vi "PH_Beckhoff_PP_PU.set RR GUI Elements to Default.vi"(0 "i ref in":refnum<vi>, 2 "PUs":T2[](array[typedef]), 5 "error in":errorcluster) -> (14 "i ref out":refnum<vi>, 19 "error out":errorcluster)   [LabVIEW 2014, in "PH_Beckhoff_PP_PU.lvlib"]
uses:
  PH_Beckhoff_PP_PU.lvlib
  PH_Basics/PH_PP_Common/PH_PP_Common.PUs.ctl
  PH_Beckhoff_PP_PU.RR Tags.ctl
  PH_Basics/PH_Common/Names/PH_Names.Subsystems.ctl
  PH_Basics/PH_PP_Common/PH_PP_Common.Devices.ctl
  PH_Basics/PH_Common/PH_Common.lvlib
  PH_Basics/PH_PP_Common/PH_PP_Common.lvlib
panel:
  in  "Ross Relais Tags":T1
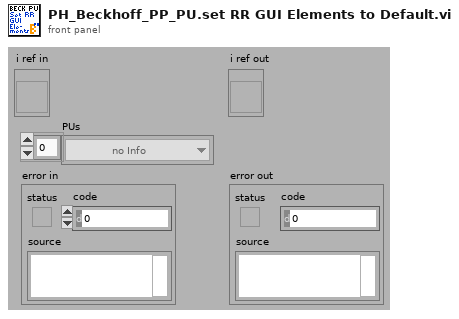
[diagram p1: front panel]
types:
  T1 = typedef "PH_Beckhoff_PP_PU.lvlib/PH_Beckhoff_PP_PU.RR Tags.ctl" = enum16{"open", "closed", "close", "Status"}
  T2 = typedef "PH_PP_Common.lvlib/PH_PP_Common.PUs.ctl" = enum16{"no Info", "PA-19mm-1", "PA-19mm-2", "PA-45mm-PILC", "PA-45mm-MAIN", "MA-PU-1", "MA-PU-2", "MA-PU-3", "MA-PU-4", "MA-PU-5", "MA-PU-6", "MA-FR", "MA-PILC", "PA-45mm-DP"}
  T3 = typedef "PH_Common.lvlib/PH_Names.Subsystems.ctl" = enum16{"no Info", "fs-FE", "ns-FE", "PA", "MA", "MAS", "COS", "Exp-LB", "Exp-LL", "PP", "PILS"}
  T4 = typedef "PH_Beckhoff_PP_PU.lvlib/PH_Beckhoff_PP_PU.i attribute.ctl" = cluster{"HV Meas":cluster{"Input GUI Ref":refnum<vi>, "Voltage Service ID":i32, "Voltage [V]":dbl, "Quality":bool, "# in Data":i32}[], "Trigger":cluster{"Status":cluster{"GUI Ref":refnum<vi>, "Status Service ID":i32, "Status":T5}, "last shot:":cluster{"GUI Ref":refnum<vi>, "Service ID":i32, "Time":string}, "DIs":cluster{"triggered":cluster{"GUI Ref":refnum<vi>, "# in Data":i32}, "fired":cluster{"GUI Ref":refnum<vi>, "# in Data":i32}}, "GUI Ref Indicator":refnum<vi>}[], "RR":cluster{"Status":cluster{"GUI Ref":refnum<vi>, "Status Service ID":i32, "Status":T5}, "DIs":cluster{"closed":cluster{"GUI Ref":refnum<vi>, "# in Data":i32}, "open":cluster{"GUI Ref":refnum<vi>, "# in Data":i32}}, "Close":cluster{"GUI Ref":refnum<vi>, "# in Data":i32}, "GUI Ref Indicator":refnum<vi>}[], "Igni":cluster{"Status":cluster{"GUI Ref":refnum<vi>, "Status Service ID":i32, "Status":T5}, "DIs":cluster{"heating on":cluster{"GUI Ref":refnum<vi>, "# in Data":i32}, "water on":cluster{"GUI Ref":refnum<vi>, "# in Data":i32}}, "Device on":cluster{"GUI Ref":refnum<vi>, "# in Data":i32}, "GUI Ref Indicator":refnum<vi>}[], "PSU":cluster{"Status":cluster{"GUI Ref":refnum<vi>, "Status Service ID":i32, "Status":T5}, "Limit Service ID":i32, "DIs":cluster{"inhibit":cluster{"GUI Ref":refnum<vi>, "# in Data":i32}, "end of charge":cluster{"GUI Ref":refnum<vi>, "# in Data":i32}, "HV on":cluster{"GUI Ref":refnum<vi>, "# in Data":i32}, "overtemp":cluster{"GUI Ref":refnum<vi>, "# in Data":i32}, "interlock":cluster{"GUI Ref":refnum<vi>, "# in Data":i32}, "load fault":cluster{"GUI Ref":refnum<vi>, "# in Data":i32}, "sum fault":cluster{"GUI Ref":refnum<vi>, "# in Data":i32}, "HV off":cluster{"GUI Ref":refnum<vi>, "# in Data":i32}, "DC ok":cluster{"GUI Ref":refnum<vi>, "# in Data":i32}}, "AIs":cluster{"voltage":cluster{"GUI Ref":refnum<vi>, "# in Data":i32}, "current":cluster{"GUI Ref":refnum<vi>, "# in Data":i32}}, "DAs":cluster{"inhibit":cluster{"GUI Ref":refnum<vi>, "# in Data":i32}, "interlock":cluster{"GUI Ref":refnum<vi>, "# in Data":i32}, "HV on":cluster{"GUI Ref":refnum<vi>, "# in Data":i32}, "Reset":cluster{"GUI Ref":refnum<vi>, "# in Data":i32}}, "AAs":cluster{"Voltage to set":cluster{"GUI Ref":refnum<vi>, "# in Data":i32}}, "GUI Ref Indicator":refnum<vi>}[], "reconfigured":cluster{"?":bool, "GUI Ref":refnum<vi>}, "PU Rack Type":T6, "HV Meas Info":T7, "PSU Info":T8}
  T5 = typedef "PH_StatusHandler.lvlib/PH_StatusHandler.Status.ctl" = i16
  T6 = typedef "PH_Beckhoff_PP_PU.lvlib/PH_Beckhoff_PP_PU.PU Rack Type.ctl" = enum16{"no Info", "PA 19mm", "PA 45mm", "MA PU 1 and 2", "MA PU 3 and 4", "MA PU 5 and 6", "MA FR and PILC"}
  T7 = typedef "PH_Beckhoff_PP_PU.lvlib/PH_Beckhoff_PP_PU.HV Meas Info.ctl" = cluster{"Period Time [s]":dbl, "Subtractor 1 [Hz]":dbl, "Devider 1 [Hz/kV]":dbl, "Subtractor 2 [Hz]":dbl, "Devider 2 [Hz/kV]":dbl}
  T8 = typedef "PH_Beckhoff_PP_PU.lvlib/PH_Beckhoff_PP_PU.PSU Info.ctl" = cluster{"Limits 1 [V]":cluster{"Lower":dbl, "Upper":dbl}, "Limits 2 [V]":cluster{"Lower":dbl, "Upper":dbl}}
  T9 = cluster{"Status":cluster{"GUI Ref":refnum<vi>, "Status Service ID":i32, "Status":T5}, "DIs":cluster{"closed":cluster{"GUI Ref":refnum<vi>, "# in Data":i32}, "open":cluster{"GUI Ref":refnum<vi>, "# in Data":i32}}, "Close":cluster{"GUI Ref":refnum<vi>, "# in Data":i32}, "GUI Ref Indicator":refnum<vi>}[]
  T10 = typedef "PH_PP_Common.lvlib/PH_PP_Common.Devices.ctl" = enum16{"no Info", "Igni", "RR", "DumpRoss", "PSU", "Trigger", "HV-Meas", "Rods", "Chiller", "Conductivity", "Mercury"}
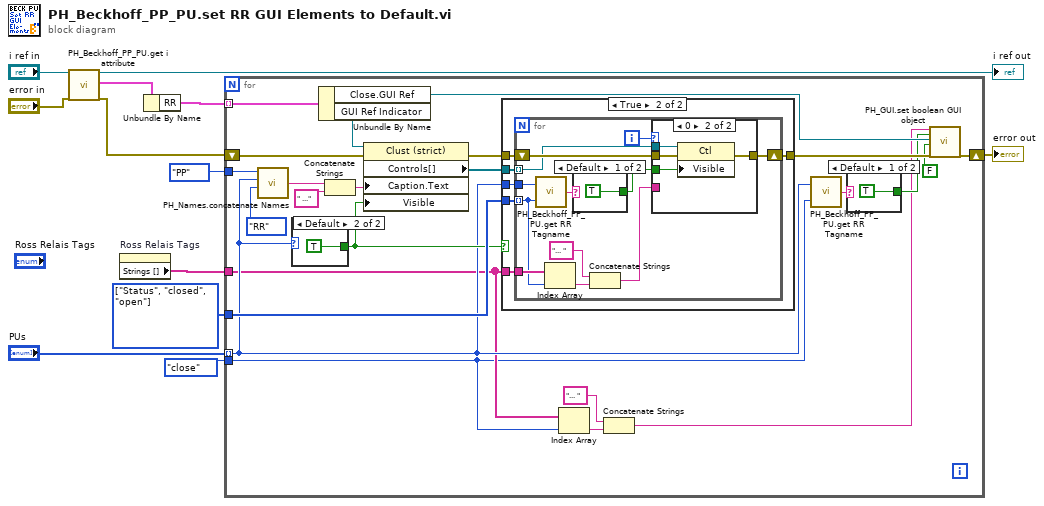
[diagram p0: block diagram]
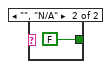
[diagram p2: hidden frame]
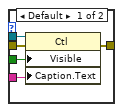
[diagram p4: hidden frame]
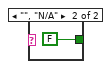
[diagram p5: hidden frame]
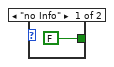
[diagram p6: hidden frame]
diagram:
  w3 = T1[] [enum."Status", enum."closed", enum."open"] items=["open", "closed", "close", "Status"]
  n1 = call "PH_Beckhoff_PP_PU.get i attribute.vi"("i ref in"="i ref in", "error in (no error)"="error in") -> ("i ref out"=→"i ref out":refnum<vi>, "i attribute"=w10:T4, "error out"=w8:errorcluster)  [unwired: 15 in]
  n2 = property on="Ross Relais Tags" class="Enum (strict)"() -> ("Strings []"=w4:string[])  [unwired: 2 in, 2 out]
  n3 = Unbundle By Name(w10) -> ("RR"=w9:T9)
  n4 = for {
    tunnel: w9 -> [w36] mode=indexing
    shift-right: [w26] -> w11
    shift-left: w8 -> [w34]
    tunnel: "PUs" -> [w16] mode=indexing
    tunnel: w3 -> [w32]
    tunnel: w4 -> [w15]
    tunnel: PH_Beckhoff_PP_PU.RR_Tags."close" ("Ross Relais Tag") -> [w13]
    tunnel: PH_Names.Subsystems."PP" ("Subsystem") -> [w20]
    n5 = call "PH_Names.concatenate Names.vi"("Devices (no info)"=PH_PP_Common.Devices."RR", "PU (no info)"=w16, "Subsystem"=w20) -> ("Subsystem_PU_Devices_Comm Type"=w21:string)  [unwired: 1 in]
    n6 = case shown="Default" w16 {
      tunnel: [FALSE TRUE] -> w30
      frame "no Info" {
      }
      frame Default {
      }
    }
    n7 = Unbundle By Name(w36) -> ("Close.GUI Ref"=w25:refnum<vi>, "GUI Ref Indicator"=w31:refnum<vi>)
    n8 = Concatenate Strings(w21, " ..." ("string")) -> (w28:string)
    n9 = property class="Clust (strict)"(reference=w31, error in=w34, "Caption.Text"=w28, "Visible"=w30) -> (error out=w35:errorcluster, "Controls[]"=w29:refnum<vi>[])  [unwired: 1 out]
    n10 = case shown="True" w30 {
      tunnel: w29 -> [_ w45]
      tunnel: w35 -> [w39 w44]
      tunnel: [w39 w43] -> w33
      tunnel: w32 -> [_ w42]
      tunnel: w16 -> [_ w41]
      tunnel: w15 -> [_ w40]
      frame False {
      }
      frame True {
        n11 = for {
          tunnel: w45 -> [w54] mode=indexing
          shift-right: [w56] -> w43
          shift-left: w44 -> [w57]
          tunnel: w41 -> [w53]
          tunnel: w42 -> [w47] mode=indexing
          tunnel: w40 -> [w55]
          i -> [w46]
          n12 = call "PH_Beckhoff_PP_PU.get RR Tagname.vi"("Ross Relais Tag"=w47, "PU"=w53) -> ("RR Tagname"=w52:string)
          n13 = Index Array(array=w55, index=w47) -> (element=w50:string)
          n14 = case shown="Default" w52 {
            tunnel: [TRUE FALSE] -> w51
            frame Default {
            }
            frame "", "N/A" {
            }
          }
          n15 = Concatenate Strings("... " ("string"), w50) -> (w49:string)
          n16 = case shown="0" w46 {
            tunnel: w57 -> [w62 w66]
            tunnel: [w61 w65] -> w56
            tunnel: w54 -> [w60 w64]
            tunnel: w51 -> [w59 w63]
            tunnel: w49 -> [w58 _]
            frame Default {
              n17 = property class="Ctl"(reference=w60, error in=w62, "Visible"=w59, "Caption.Text"=w58) -> (error out=w61:errorcluster)  [unwired: 1 out]
            }
            frame 0 {
              n18 = property class="Ctl"(reference=w64, error in=w66, "Visible"=w63) -> (error out=w65:errorcluster)  [unwired: 1 out]
            }
          }
        }
      }
    }
    n19 = Index Array(array=w15, index=w13) -> (element=w18:string)
    n20 = Concatenate Strings("... " ("string"), w18) -> (w14:string)
    n21 = call "PH_Beckhoff_PP_PU.get RR Tagname.vi"("Ross Relais Tag"=w13, "PU"=w16) -> ("RR Tagname"=w23:string)
    n22 = case shown="Default" w23 {
      tunnel: [TRUE FALSE] -> w22
      frame Default {
      }
      frame "", "N/A" {
      }
    }
    n23 = call "PH_GUI.set boolean GUI object.vi"("Caption"=w14, "Visible (true)"=w22, "Boolean Knob GUI Ref"=w25, "Value"=FALSE, "error in (no error)"=w33) -> ("error out"=w26:errorcluster)  [unwired: 14 in]
  }
  "error out" <- w11
